vi "N5232-PNA_ExecuteShortcut.vi"(0 "Session In":refnum<visa-resource-name>="TCPIP0::169.254.70.180::inst0::INSTR", 11 "error in":errorcluster {"code" format="%.0x"}, 13 "ShortcutNum":string) -> (4 "Session Out":refnum<visa-resource-name>="TCPIP0::169.254.70.180::inst0::INSTR", 15 "error out":errorcluster {"code" format="%.0x"})   [LabVIEW 2018]
doc: "Launches the Instrument I/O Assistant, which you can use to communicate with message-based instruments and graphically parse the response. For example you can communicate with an instrument that uses a serial, Ethernet, or GPIB interface."
panel:
  # "Shortcuts on N5232A are also known as \"Macros\" listed in the UTILITY menu"
  # "Enter a number 1-25. Leave Blank or write \"ALL\" to get the list of all available shortcuts"
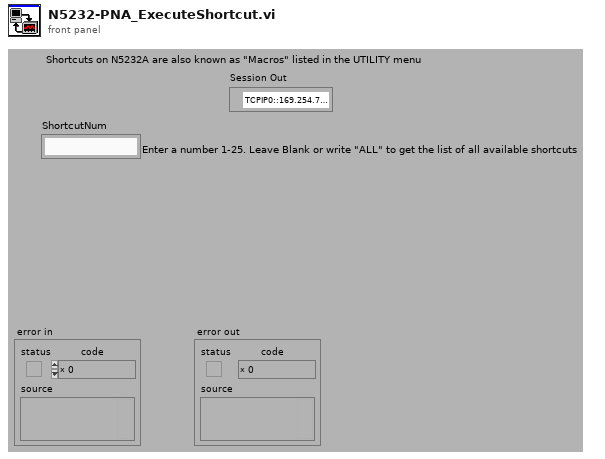
[diagram p1: front panel]
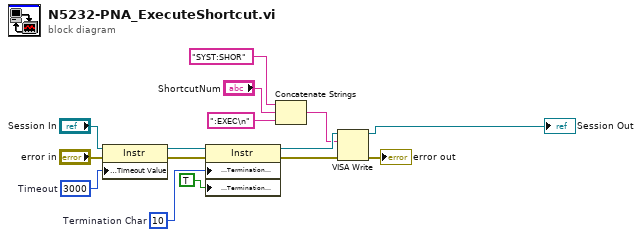
[diagram p0: block diagram]
diagram:
  w10 = u8 10  # Termination Char
  w15 = u32 3000  # Timeout
  n1 = property class="Instr"(reference="Session In", error in="error in", "General Settings:Timeout Value"=w15) -> (reference out=w9:refnum<visa-resource-name>, error out=w12:errorcluster)
  n2 = property class="Instr"(reference=w9, error in=w12, "Message Based Settings:Termination Character"=w10, "Message Based Settings:Termination Character Enable"=TRUE ("enable")) -> (reference out=w7:refnum<visa-resource-name>, error out=w11:errorcluster)
  n3 = Concatenate Strings("SYST:SHOR" ("Command"), "ShortcutNum", ":EXEC\n" ("Command")) -> (w6:string)
  n4 = VISA Write(VISA resource name=w7, write buffer=w6, error in (no error)=w11) -> (VISA resource name out=→"Session Out":refnum<visa-resource-name>, error out=→"error out":errorcluster)  [unwired: 1 out]
